vi "uTTA_CloseCOM.vi"() -> ()   [LabVIEW 2021]
panel:
  in  "VISA resource name":refnum<visa-resource-name>
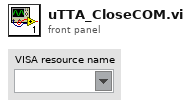
[diagram p1: front panel]
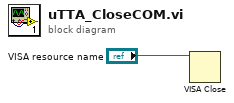
[diagram p0: block diagram]
diagram:
  n1 = VISA Close(VISA resource name="VISA resource name") -> ()  [unwired: 1 in, 1 out]
